vi "pwm_values_to_motor_cmds.vi"(8 "Old rudder cmd":T1 min=-0.95 max=0.95 scale=1.0..-1.0, 9 "Old sail cmd":dbl, 10 "Rudder duty cycle fraction":dbl, 11 "Sail duty cycle fraction":dbl) -> (2 "Rudder cmd OUT":T1 min=-0.95 max=0.95 scale=1.0..-1.0, 3 "Sail cmd OUT":dbl)   [LabVIEW 2013]
doc: "This VI takes in PWM values read off the FPGA and converts them to useable commands for the sails and rudder."
uses:
  Data/TypeDefs/Rudder Set Suggestions.ctl
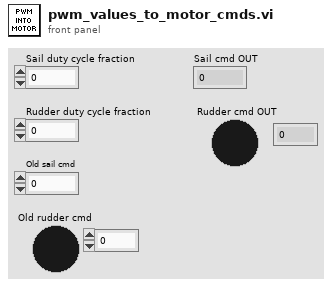
[diagram p1: front panel]
types:
  T1 = typedef "Rudder Set Suggestions.ctl" = dbl
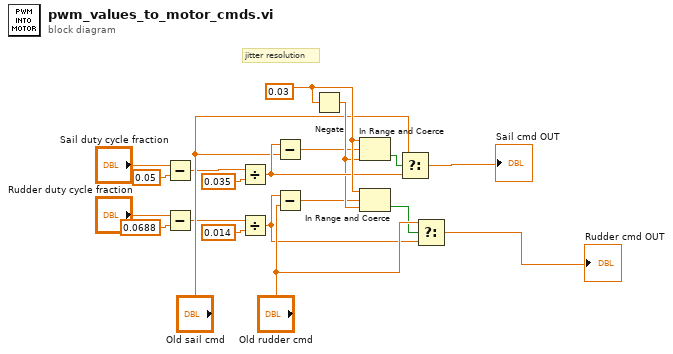
[diagram p0: block diagram]
diagram:
  w20 = 0.03 ("Jitter cutout")
  # "jitter resolution"
  n1 = Subtract(x="Sail duty cycle fraction", y=0.05) -> (x-y=w3:dbl)
  n2 = Subtract(x="Rudder duty cycle fraction", y=0.0688) -> (x-y=w6:dbl)
  n3 = Divide(x=w3, y=0.035) -> (x/y=w19:dbl)
  n4 = Divide(x=w6, y=0.014) -> (x/y=w14:dbl)
  n5 = Subtract(x=w19, y="Old sail cmd") -> (x-y=w9:dbl)
  n6 = Subtract(x=w14, y="Old rudder cmd") -> (x-y=w12:T1)
  n7 = Negate(x=w20) -> (-x=w18:dbl)
  n8 = In Range and Coerce(upper limit=w20, x=w9, lower limit=w18) -> (In Range?=w10:bool)  [unwired: 1 out]
  n9 = In Range and Coerce(upper limit=w20, x=w12, lower limit=w18) -> (In Range?=w13:bool)  [unwired: 1 out]
  n10 = Select(t="Old sail cmd", s=w10, f=w19) -> (s? t:f=→"Sail cmd OUT":dbl)
  n11 = Select(t="Old rudder cmd", s=w13, f=w14) -> (s? t:f=→"Rudder cmd OUT":T1)
